vi "Wait for Signal.vi"(4 "Error In":errorcluster, 7 "Timeout":dbl[unit]=10.0) -> (0 "Error Out":errorcluster)   [LabVIEW 2015, in "not_Launch Completed.lvlib"]
uses:
  not_Launch Completed.lvlib
  <vilib>/Utility/error.llb/Error Cluster From Error Code.vi
  <vilib>/ErrorRing/Error Ring.xnode
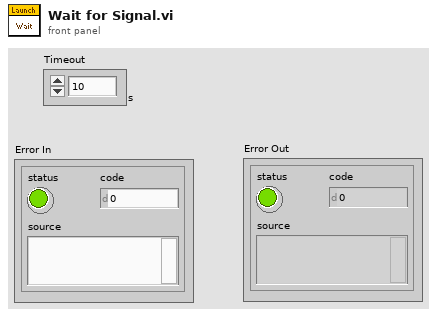
[diagram p1: front panel]
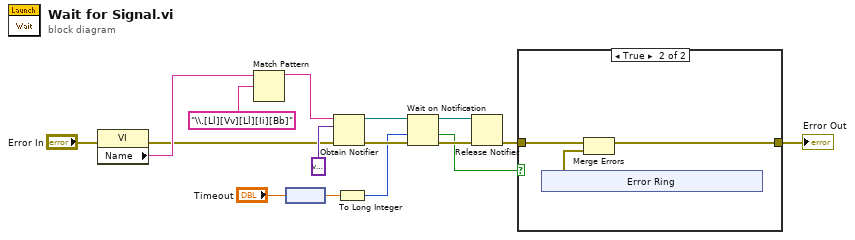
[diagram p0: block diagram]
diagram:
  n1 = property class="VI"(error in="Error In") -> (error out=w1:errorcluster, "Name"=w5:string)  [unwired: 1 in, 1 out]
  n2 = Match Pattern(string=w5, regular expression="\\.[Ll][Vv][Ll][Ii][Bb]") -> (before substring=w3:string)  [unwired: 1 in, 3 out]
  n3 = node("Timeout") -> (w10:dbl)
  n4 = Obtain Notifier(name (unnamed)=w3, notification data type=variant ("element data type"), error in (no error)=w1) -> (notifier out=w15:refnum<notifier>, error out=w16:errorcluster)  [unwired: 1 in, 1 out]
  n5 = To Long Integer(number=w10) -> (32bit integer=w9:i32)
  n6 = Wait on Notification(notifier=w15, timeout in ms (-1)=w9, error in (no error)=w16) -> (notifier out=w14:refnum<notifier>, timed out?=w8:bool, error out=w13:errorcluster)  [unwired: 1 in, 1 out]
  n7 = Release Notifier(notifier=w14, error in (no error)=w13) -> (error out=w7:errorcluster)  [unwired: 1 in, 2 out]
  n8 = case shown="True" w8 {
    tunnel: w7 -> [w17 w20]
    tunnel: [w17 w19] -> w6
    frame False {
    }
    frame True {
      n9 = xnode "Error Ring"() -> ("error out"=w18:errorcluster)
      n10 = Merge Errors(w20, w18) -> (w19:errorcluster)
    }
  }
  "Error Out" <- w6
